vi "ShowResultUsingSP.vi"() -> ()   [LabVIEW 2019]
uses:
  <vilib>/addons/database/Connection.llb/DB Tools Open Connec (String).vi
  <vilib>/addons/database/Connection.llb/Conn Execute.vi
  <vilib>/addons/database/Recordset.llb/Rec Fetch Recordset Data (R).vi
  <vilib>/addons/database/Recordset.llb/Rec Destroy - Connection.vi
  <vilib>/addons/database/_DB Variant To Data/Database Variant To Data.xnode
  <vilib>/addons/database/NI_Database_API.lvlib
panel:
  out "OutPut":string[][](array[string])
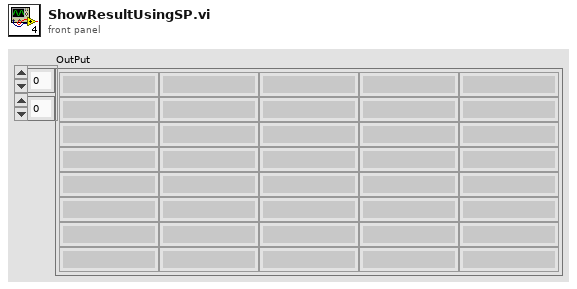
[diagram p1: front panel]
types:
  T1 = typedef "NI_Database_API.lvlib/Conn ObjectReference.ctl" = refnum<k1>
  T2 = typedef "NI_Database_API.lvlib/Rec ObjectReference.ctl" = refnum<k1>
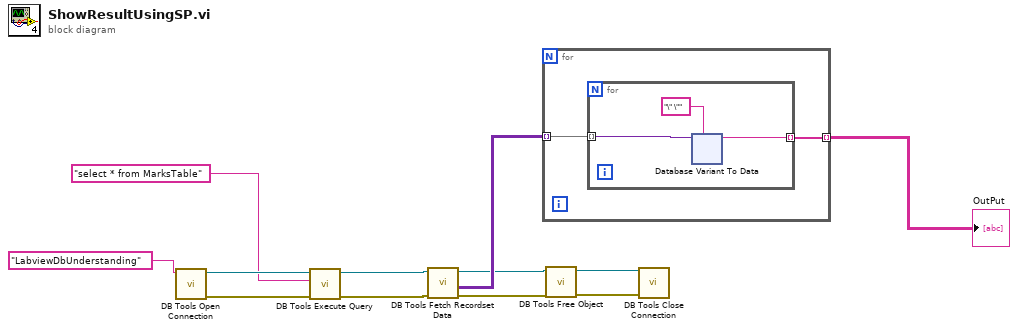
[diagram p0: block diagram]
diagram:
  n1 = call-poly <vilib>:"DB Tools Open Connection.vi"("connection information"="LabviewDbUnderstanding") -> ("error out"=w10:errorcluster, "connection reference"=w11:T1)  [unwired: 7 in]
  n2 = call-poly <vilib>:"DB Tools Execute Query.vi"("error in (no error)"=w10, "SQL query"="select * from MarksTable", "connection reference"=w11) -> ("error out"=w7:errorcluster, "recordset reference"=w8:T2)  [unwired: 5 in]
  n3 = call-poly <vilib>:"DB Tools Fetch Recordset Data.vi"("error in (no error)"=w7, "recordset reference"=w8) -> ("error out"=w3:errorcluster, "recordset data"=w6:variant[][], "recordset reference out"=w4:T2)  [unwired: 3 in]
  n4 = for {
    tunnel: w6 -> [w14] mode=indexing
    tunnel: [w13] -> w5 mode=indexing
    n5 = for {
      tunnel: w14 -> [w17] mode=indexing
      tunnel: [w15] -> w13 mode=indexing
      n6 = xnode "Database Variant To Data"("database variant"=w17, "type"="\" \"") -> ("data"=w15:string)  [unwired: 1 in, 1 out]
    }
  }
  "OutPut" <- w5
  n7 = call-poly <vilib>:"DB Tools Free Object.vi"("error in (no error)"=w3, "recordset reference"=w4) -> ("error out"=w1:errorcluster, "connection reference"=w2:T1)  [unwired: 8 in]
  n8 = call <vilib>:"DB Tools Close Connection.vi"("error in (no error)"=w1, "connection reference"=w2) -> ()  [unwired: 5 in, 1 out]
